vi "Solve1.vi"(8 "Error In":errorcluster, 11 "object in":refnum<class "2024_10.lvclass">) -> (0 "Error Out":errorcluster, 2 "Result":u64, 3 "object out":refnum<class "2024_10.lvclass">)   [LabVIEW 2023, in "2024_10.lvclass"]
uses:
  2024_10.lvclass
  2024_10.lvclass/2024_10.ctl
  8882d225-cd61-4e30-955f-a4d2e3f62846.vi
panel:
  out "TrailHead":cluster{i32, i32}[](array[cluster])
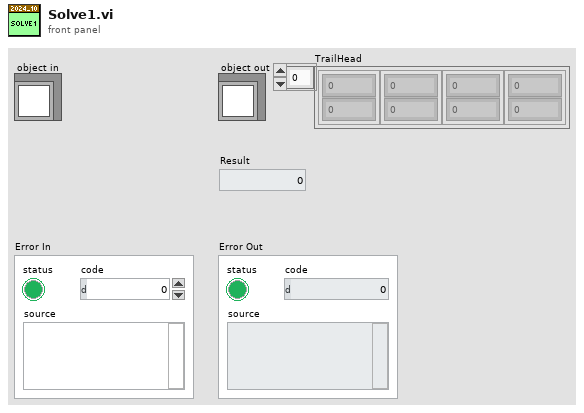
[diagram p1: front panel]
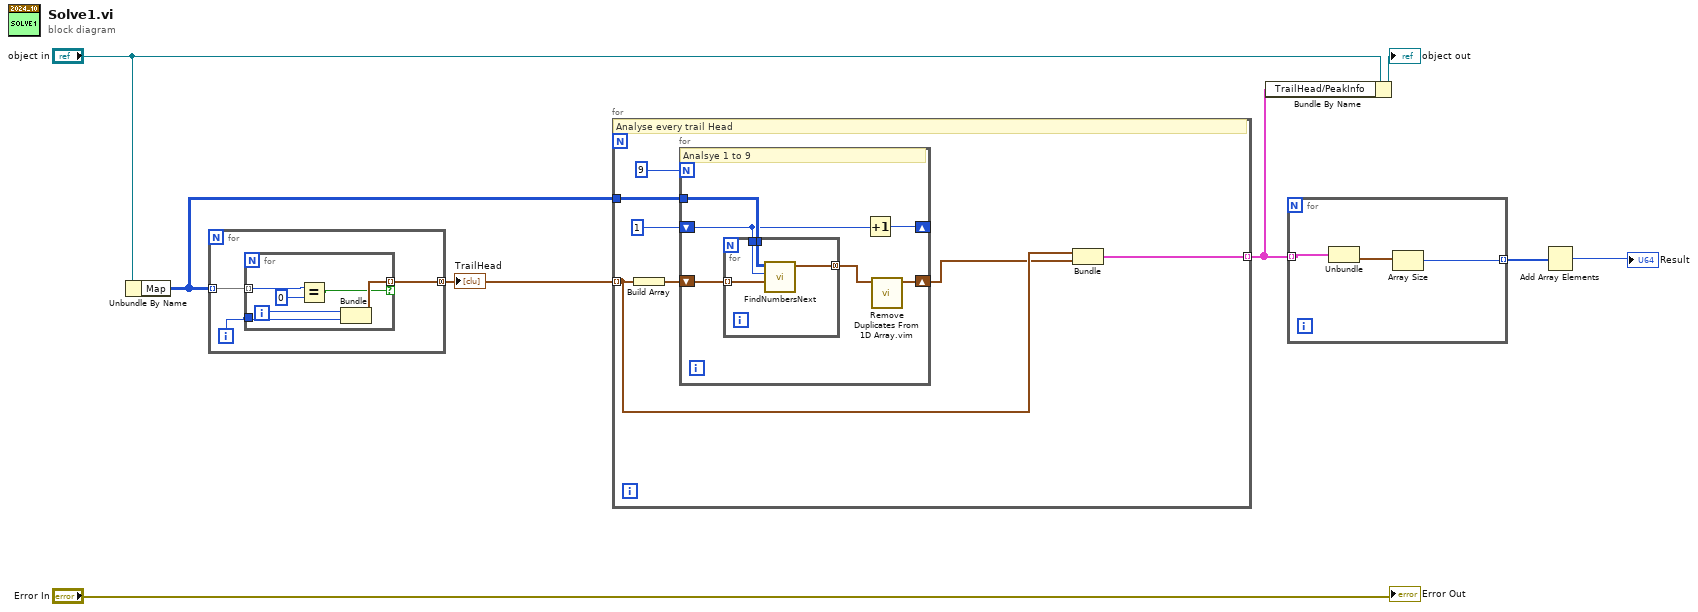
[diagram p0: block diagram]
diagram:
  n1 = Unbundle By Name("object in") -> ("Map"=w5:u8[][])
  n2 = for {
    tunnel: w5 -> [w11] mode=indexing
    tunnel: [w9] -> w6 mode=concatenating
    i -> [w10]
    n3 = for {
      tunnel: w11 -> [w17] mode=indexing
      tunnel: w10 -> [w14]
      tunnel: [w13] -> w9 mode=indexing if=w12
      i -> [w15]
      n4 = Equal?(x=w17, y=u8 0) -> (x = y?=w12:bool)
      n5 = Bundle(w15, w14) -> (w13:cluster{i32, i32})  [unwired: 1 in]
    }
  }
  "TrailHead" <- w6
  n6 = for {
    tunnel: w6 -> [w22] mode=indexing
    tunnel: w5 -> [w24]
    tunnel: [w20] -> w1 mode=indexing
    # "Analyse every trail Head"
    n7 = Build Array(w22) -> (w23:cluster{i32, i32}[])
    n8 = for {
      N: u8 9 ("y") -> [_]
      tunnel: w24 -> [w29]
      shift-right: [w26] -> _
      shift-left: u8 1 ("y") -> [w27]
      shift-right: [w25] -> w21
      shift-left: w23 -> [w30]
      # "Analsye 1 to 9"
      n9 = for {
        tunnel: w30 -> [w34] mode=indexing
        tunnel: w29 -> [w33]
        tunnel: w27 -> [w32]
        tunnel: [w31] -> w28 mode=concatenating
        n10 = call "FindNumbersNext.vi"("Cluster"=w34, "Numeric"=w32, "Map"=w33) -> ("Array"=w31:cluster{"Numeric":i32, "Numeric":i32}[])  [unwired: 8 in]
      }
      n11 = Increment(x=w27) -> (x+1=w26:u8)
      n12 = call "Remove Duplicates From 1D Array.vim"("array"=w28) -> ("array with duplicates removed"=w25:cluster{"Numeric":i32, "Numeric":i32}[])  [unwired: 10 in]
    }
    n13 = Bundle(w22, w21) -> (w20:cluster{cluster{i32, i32}, cluster{i32, i32}[]})  [unwired: 1 in]
  }
  n14 = Bundle By Name(cluster="object in", "TrailHead/PeakInfo"=w1) -> (→"object out":refnum<class "2024_10.lvclass">)
  n15 = for {
    tunnel: w1 -> [w37] mode=indexing
    tunnel: [w35] -> w4 mode=indexing
    n16 = Unbundle(w37) -> (w36:cluster{i32, i32}[])  [unwired: 1 out]
    n17 = Array Size(array=w36) -> (size(s)=w35:i32)
  }
  n18 = Add Array Elements(numeric array=w4) -> (sum=→"Result":i32)
  "Error Out" <- "Error In"
